vi "Set tab pages name.vi"(9 "Array":string[][](array[string]), 10 "Numeric":i32, 11 "Control in":refnum<vi>) -> (0 "error out":errorcluster, 3 "Control OUT":refnum<vi>)   [LabVIEW 2016]
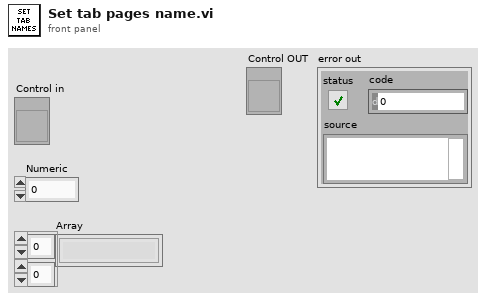
[diagram p1: front panel]
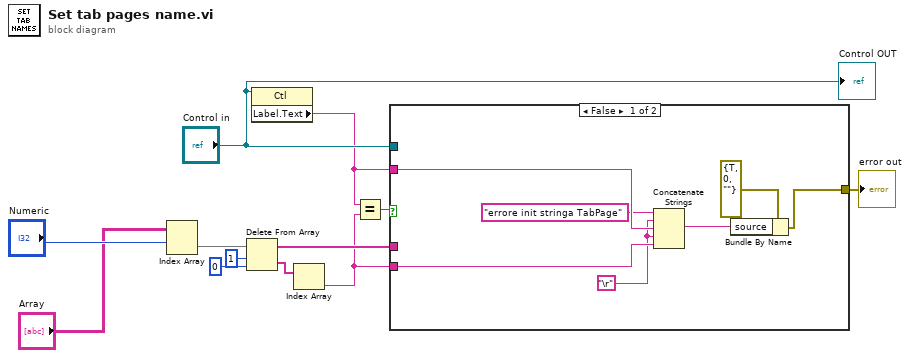
[diagram p0: block diagram]
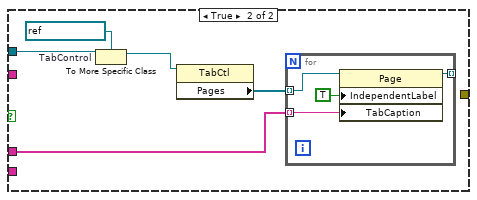
[diagram p2: hidden frame]
diagram:
  n1 = Index Array(array="Array", index (row)="Numeric") -> (element=w9:string[])  [unwired: 1 in]
  n2 = Delete From Array(array=w9, length=1, index=0) -> (deleted portion=w5:string[], array with subset deleted=w12:string[])
  n3 = property class="Ctl"(reference="Control in") -> ("Label.Text"=w2:string)  [unwired: 1 in, 2 out]
  n4 = Index Array(array=w5) -> (element=w1:string)  [unwired: 1 in]
  n5 = Equal?(x=w2, y=w1) -> (x = y?=w4:bool)
  n6 = case shown="False" w4 {
    tunnel: w12 -> [_ w24]
    tunnel: "Control in" -> [_ w20]
    tunnel: [w18 _] -> w3
    tunnel: w2 -> [w17 _]
    tunnel: w1 -> [w16 _]
    frame False {
      w13 = "\r"
      n7 = Concatenate Strings("errore init stringa TabPage" ("string"), w13, w17, w13, w16) -> (w14:string)
      n8 = Bundle By Name(cluster=errorcluster {"status"=TRUE, "code"=0, "source"=""} ("error out"), "source"=w14) -> (w18:errorcluster)
    }
    frame True {
      w21 = refnum<vi> refnum  # TabControl
      n9 = To More Specific Class(target class=w21, reference=w20) -> (specific class reference=w22:refnum<vi>)  [unwired: 1 in, 1 out]
      n10 = property class="TabCtl"(reference=w22) -> ("Pages"=w23:refnum<vi>[])  [unwired: 1 in, 2 out]
      n11 = for {
        tunnel: w23 -> [w28] mode=indexing
        tunnel: w24 -> [w27] mode=indexing
        tunnel: [w25] -> _ mode=indexing
        n12 = property class="Page"(reference=w28, "IndependentLabel"=TRUE ("Independent Label"), "TabCaption"=w27) -> (reference out=w25:refnum<vi>)  [unwired: 1 in, 1 out]
      }
    }
  }
  "error out" <- w3
  "Control OUT" <- "Control in"
